vi "GlobalGetBeamDiagnosticOnOff.vi"() -> ()   [LabVIEW 2011]
panel:
  out "GetBeamDiagnistic":bool
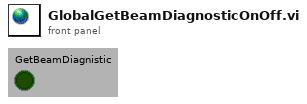
[diagram p1: front panel]
diagram:
